vi "Send.vi"(5 "Topic Broadcast?":bool, 7 "Message Priority":T1, 8 "error in (no error)":errorcluster, 9 "Timeout":i32, 10 "Message":refnum<class "Message Interface.lvclass">, 11 "Message Transport Singleton in":refnum<class "Message Transport Singleton.lvclass">=refnum) -> (0 "error out":errorcluster, 2 "Timed Out?":bool, 3 "Message Transport Singleton out":refnum<class "Message Transport Singleton.lvclass">)   [LabVIEW 2016, in "Stream Mediator.lvlib" / "Message Transport Singleton.lvclass"]
doc: "--\nCopyright © 2017 Composed SystemsI All rights reserved.\n\nAuthor: Jon McBee <jon.mcbee@composed.io>\n\nThis library is provided \"AS IS\" ,WITHOUT WARRANTIES OR\nCONDITIONS OF ANY KIND, either express or implied.\n\nComposed Systems -- composed.io\n\nStream 0.0.1.1\nJon McBee - Composed Systems\nCopyright (c) 2017, Composed Systems"
uses:
  <userlib>/Composed Systems/Stream/Mediator/Classes/Message Transport Singleton/Message Transport Singleton.lvclass
  C:/Program Files (x86)/National Instruments/LabVIEW 2016/user.lib/Composed Systems/Stream/Mediator/Classes/Message Transport Interface/Message Transport Interface.lvclass
  <userlib>/Composed Systems/Stream/Mediator/Classes/Message Interface/Message Interface.lvclass
  <userlib>/Composed Systems/Stream/Mediator/Classes/Message Transport Interface/Message Priority.ctl
  <userlib>/Composed Systems/Stream/Mediator/Classes/Message Interface/Message Interface.lvclass/Message Interface.ctl
  <userlib>/Composed Systems/Stream/Mediator/Classes/Message Transport Singleton/Message Transport Singleton.lvclass/Message Transport Singleton.ctl
  <userlib>/Composed Systems/Stream/Mediator/Classes/Message Transport Interface/Message Transport Interface.lvclass
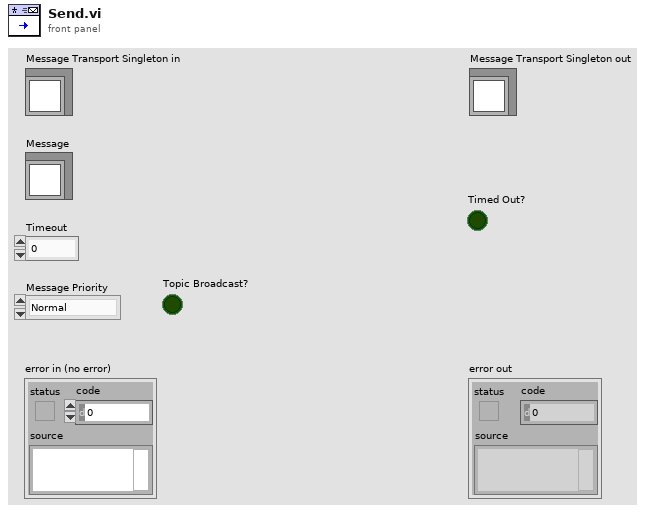
[diagram p1: front panel]
types:
  T1 = typedef "Stream Mediator.lvlib/Message Transport Interface.lvclass/Message Priority.ctl" = enum16{"Normal", "High"}
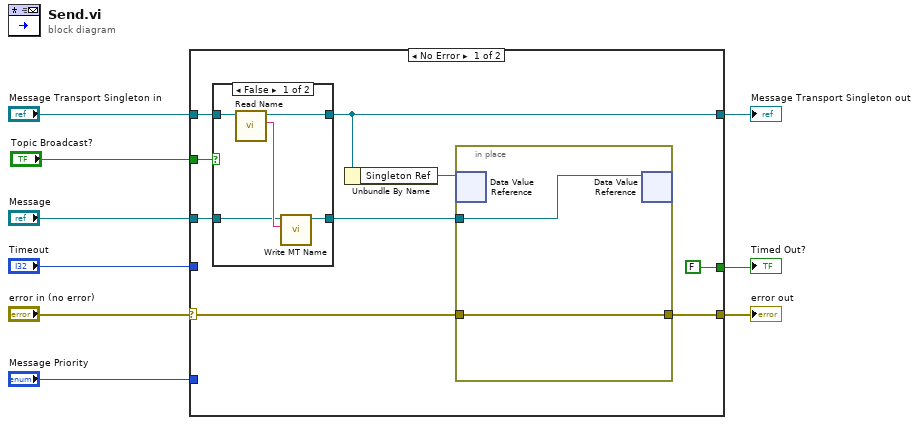
[diagram p0: block diagram]
diagram:
  n1 = case shown="No Error" "error in (no error)" {
    selector: "error in (no error)" -> [w17 w29]
    tunnel: [w16 w29] -> w8
    tunnel: "Message Priority" -> [_ _]
    tunnel: [w13 w28] -> w6
    tunnel: "Message Transport Singleton in" -> [w14 w28]
    tunnel: "Message" -> [w12 _]
    tunnel: "Timeout" -> [_ _]
    tunnel: [FALSE _] -> w2
    tunnel: "Topic Broadcast?" -> [w10 _]
    frame No Error {
      n2 = case shown="False" w10 {
        tunnel: w14 -> [w22 w25]
        tunnel: [w21 w25] -> w13
        tunnel: w12 -> [w20 w24]
        tunnel: [w19 w24] -> w11
        frame False {
          n3 = call <userlib>:"Read Name.vi"("Message Transport Interface in"=w22) -> ("Name"=w23:string, "Message Transport Interface out"=w21:refnum<class "Message Transport Singleton.lvclass">)  [unwired: 8 in, 1 out]
          n4 = call <userlib>:"Write MT Name.vi"("MT Name"=w23, "Message Interface in"=w20) -> ("Message Interface out"=w19:refnum<class "Message Interface.lvclass">)  [unwired: 9 in]
        }
        frame True {
        }
      }
      n5 = Unbundle By Name(w13) -> ("Singleton Ref"=w18:refnum<data-value>)
      n6 = in-place {
        in-place-border: [w27] -> w16
        in-place-border: w17 -> [w27]
        in-place-border: w11 -> [w26]
        n7 = in-place-dvr #1(w18) -> ()  [unwired: 2 out]
        n8 = in-place-dvr #1(w26) -> ()  [unwired: 2 out]
      }
    }
    frame Error {
    }
  }
  "error out" <- w8
  "Message Transport Singleton out" <- w6
  "Timed Out?" <- w2
